vi "Initialize New Motor.vi"() -> ()   [LabVIEW 2014]
uses:
  ALPHA5 RS485/typedefs/Port Selection Info.ctl
  ALPHA5 RS485/ALPHA5 RS485.lvlib
panel:
  out "Failed Params":u16[](array[numeric]) format="%.0x"
  out "error out":errorcluster
  in  "error in (no error)":errorcluster caption="error in"
  in  "Port Selection Info In":T1={"Port Name"="COM5", "Amplifier Num"=1, "Baud Rate"=38400, "Char Formation"=enum."0"} {"Baud Rate" items=["38400"=38400, "19200"=19200, "9600"=9600, "115200"=0]; "Amplifier Num" max=31}
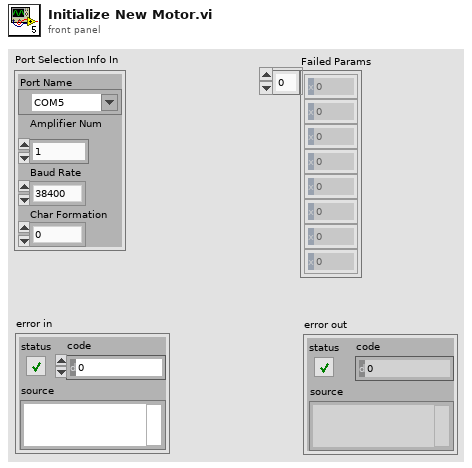
[diagram p1: front panel]
types:
  T1 = typedef "ALPHA5 RS485.lvlib/Port Selection Info.ctl" = cluster{"Port Name":refnum<visa-resource-name>, "Amplifier Num":u8, "Baud Rate":u32, "Char Formation":enum16{"0", "1", "2", "3", "4", "5"}}
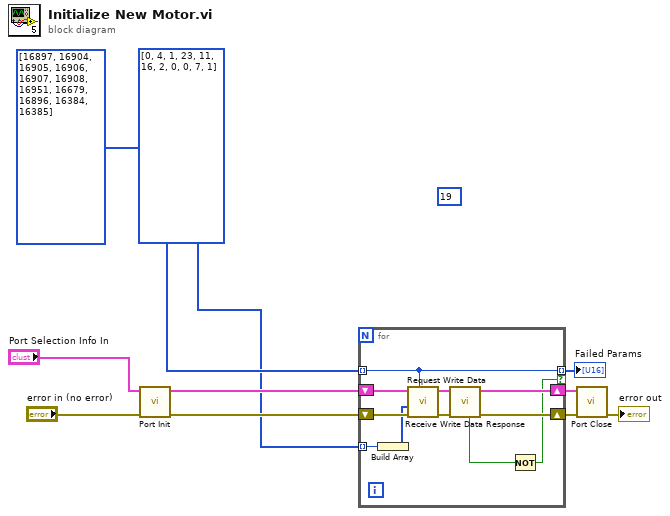
[diagram p0: block diagram]
diagram:
  (unwired) 19
  n1 = call "Port Init.vi"("error in (no error)"="error in (no error)", "Port Selection Info In"="Port Selection Info In") -> ("error out"=w8:errorcluster, "Port Selection Info Out"=w9:T1)  [unwired: 8 in]
  n2 = for {
    shift-right: [w17] -> w6
    shift-left: w9 -> [w21]
    shift-right: [w16] -> w5
    shift-left: w8 -> [w20]
    tunnel: u16[] [16897, 16904, 16905, 16906, 16907, 16908, 16951, 16679, 16896, 16384, 16385] -> [w13] mode=indexing
    tunnel: i32[] [0, 4, 1, 23, 11, 16, 2, 0, 0, 7, 1] ("Data") -> [w15] mode=indexing
    tunnel: [w13] -> w2 mode=indexing if=w11
    n3 = Build Array(w15) -> (w14:i32[])
    n4 = call "Request Write Data.vi"("Address"=w13, "error in (no error)"=w20, "Data"=w14, "Port Selection Info"=w21) -> ("error out"=w18:errorcluster, "Port Selection Info Out"=w19:T1)  [unwired: 5 in, 1 out]
    n5 = call "Receive Write Data Response.vi"("error in (no error)"=w18, "Port Selection Info"=w19) -> ("error out"=w16:errorcluster, "Port Selection Info Out"=w17:T1, "CRC Match"=w12:bool)  [unwired: 3 in, 4 out]
    n6 = Not(x=w12) -> (.not. x?=w11:bool)
  }
  "Failed Params" <- w2
  n7 = call "Port Close.vi"("error in (no error)"=w5, "Port Selection Info In"=w6) -> ("error out"=→"error out":errorcluster)  [unwired: 9 in]
